vi "Write--clear.vi"(8 "error in (no error)":errorcluster, 11 "VISA resource name":refnum<visa-resource-name>) -> (0 "error out":errorcluster, 2 "Comando(string)":string, 3 "VISA resource name out":refnum<visa-resource-name>)   [LabVIEW 2020, in "Control de MaP.lvlib"]
doc: "convierte la selección de comando a cadena y lo envía al puerto seleccionado"
uses:
  Control de MaP.lvlib
  <vilib>/Instr/_visa.llb/VISA Flush IO Buffer Mask.ctl
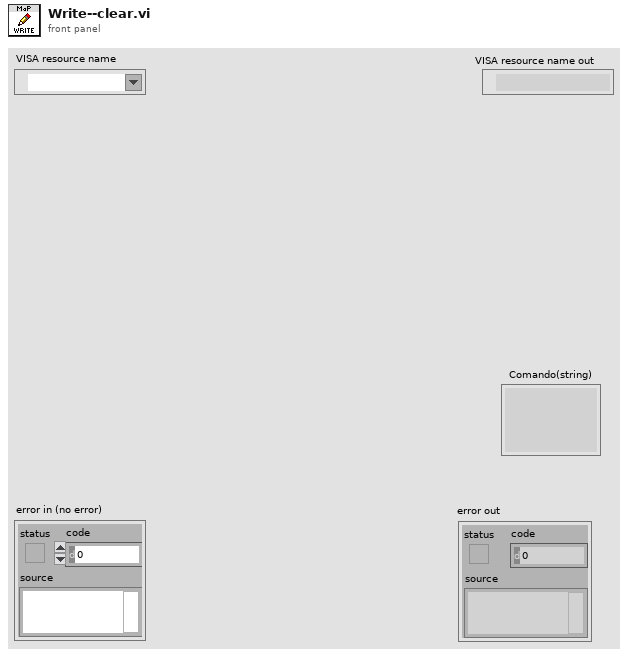
[diagram p1: front panel]
types:
  T1 = typedef "VISA Flush IO Buffer Mask.ctl" = u16
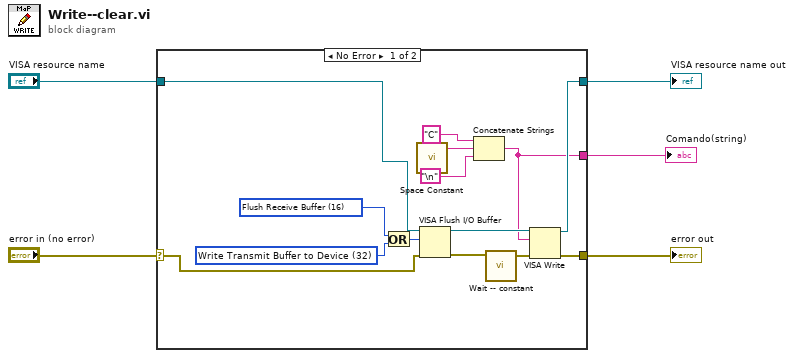
[diagram p0: block diagram]
diagram:
  n1 = case shown="No Error" "error in (no error)" {
    selector: "error in (no error)" -> [w13 w21]
    tunnel: "VISA resource name" -> [w12 w20]
    tunnel: [w19 w20] -> w4
    tunnel: [w18 w21] -> w2
    tunnel: [w16 _] -> w1
    frame No Error {
      w10 = T1 32 items=["Flush Receive Buffer"=16, "Write Transmit Buffer to Device"=32, "Flush Receive Buffer (No I/O)"=64, "Flush Transmit Buffer"=128] ("Mask")
      w11 = T1 16 items=["Flush Receive Buffer"=16, "Write Transmit Buffer to Device"=32, "Flush Receive Buffer (No I/O)"=64, "Flush Transmit Buffer"=128] ("Mask")
      n2 = Or(x=w11, y=w10) -> (x .or. y?=w9:T1)
      n3 = call <vilib>:"Space Constant.vi"() -> ("String"=w6:string)
      n4 = VISA Flush I/O Buffer(VISA resource name=w12, mask (16)=w9, error in (no error)=w13) -> (VISA resource name out=w17:refnum<visa-resource-name>, error out=w15:errorcluster)
      n5 = Concatenate Strings("C" ("string"), w6, "\n") -> (w16:string)
      n6 = call "Wait -- constant.vi"("error in (no error)"=w15) -> ("error out"=w14:errorcluster)  [unwired: 6 in]
      n7 = VISA Write(VISA resource name=w17, write buffer=w16, error in (no error)=w14) -> (VISA resource name out=w19:refnum<visa-resource-name>, error out=w18:errorcluster)  [unwired: 1 out]
    }
    frame Error {
    }
  }
  "VISA resource name out" <- w4
  "error out" <- w2
  "Comando(string)" <- w1
